vi "WPI_CameraGet Image Data String.vi"(8 "error in (no error)":errorcluster, 11 "CameraDevRef":T1) -> (0 "error out":errorcluster, 2 "Image Data String":string, 3 "CameraDevRef Out":T1)   [LabVIEW 2017]
doc: "Returns a JPEG file as a string, which is useful for saving images to disk. Use the Start VI to start acquiring image data from the camera before you use the Get Image Data String VI to retrieve an image. When you run this VI, this VI retrieves the most current snapshot of the image data from the camera.\n\nThis software is licensed. Open the labview\\readme\\WPI Robotics Library Open Source License.txt file for more information."
uses:
  <vilib>/Rock Robotics/WPI/Camera/WPI_CameraDevRef.ctl
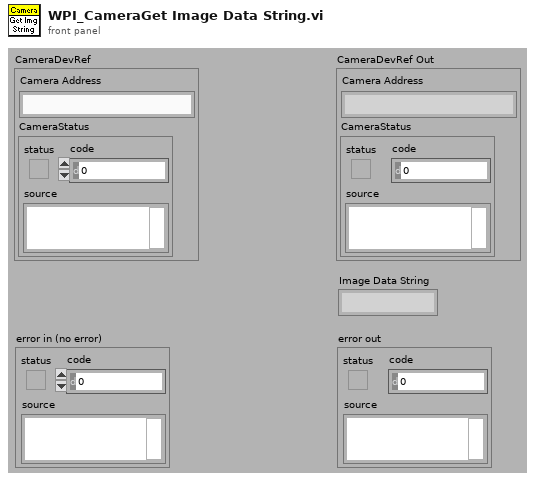
[diagram p1: front panel]
types:
  T1 = typedef "WPI_CameraDevRef.ctl" = cluster{"Camera Address":string, "CameraStatus":errorcluster}
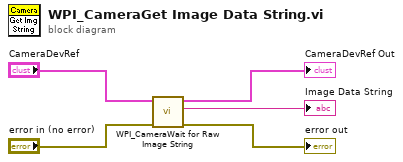
[diagram p0: block diagram]
diagram:
  n1 = call <vilib>:"WPI_CameraWait for Raw Image String.vi"("error in (no error)"="error in (no error)", "CameraDevRef"="CameraDevRef") -> ("error out"=→"error out":errorcluster, "String"=→"Image Data String":string, "CameraDevRef Out"=→"CameraDevRef Out":T1)  [unwired: 1 in, 6 out]
